vi "Get Subpanel Ref.vi"(8 "error in (no error)":errorcluster, 11 "Scan SBlock in":refnum<class "Scan SBlock.lvclass">) -> (0 "error out":errorcluster, 2 "vi reference":refnum<vi>, 3 "Scan SBlock out":refnum<class "Scan SBlock.lvclass">)   [LabVIEW 2020, in "TALOS.lvlib" / "Run Utilities.lvlib" / "Scan SBlock.lvclass"]
uses:
  Scan SBlock.lvclass
  Scan SBlock.lvclass/Scan SBlock.ctl
  Scan Mode Panel.vi
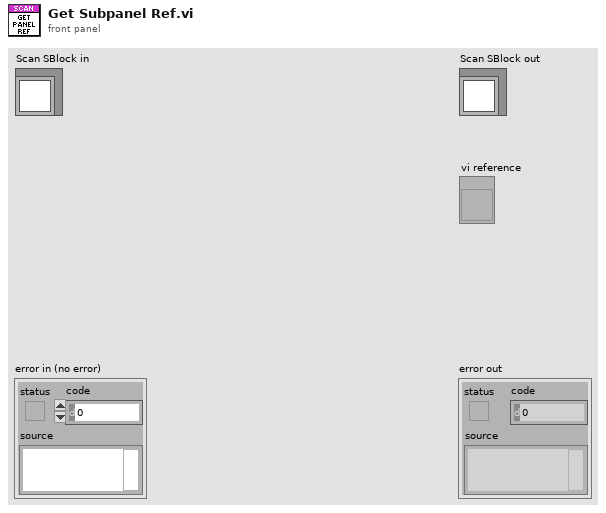
[diagram p1: front panel]
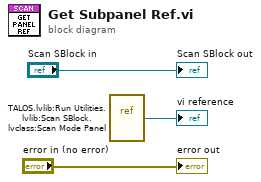
[diagram p0: block diagram]
diagram:
  n1 = vi-ref "TALOS.lvlib:Run Utilities.lvlib:Scan SBlock.lvclass:Scan Mode Panel.vi"() -> (→"vi reference":refnum<vi>)
  "error out" <- "error in (no error)"
  "Scan SBlock out" <- "Scan SBlock in"
